vi "TicTacToe.vi"() -> ()   [LabVIEW 2018]
panel:
  out "Human Win":dbl
  in  "Show XO plate":bool
  out "Computer Win":dbl
  out "Tie":bool
  out "No one Won":bool
  out "Game Over":bool
  out "Computer Won":bool
  out "Human Won":bool
  out "Turn":string
  out "XO array":string[][](array[string])
  in  "START GAME":bool
  in  "Boolean 9":bool
  in  "Boolean 8":bool
  in  "Boolean 7":bool
  in  "Boolean 6":bool
  in  "Boolean 5":bool
  in  "Boolean 4":bool
  in  "Boolean 3":bool
  in  "Boolean 2":bool
  in  "Boolean":bool
  in  "STOP GAME":bool
  in  "Turn":bool
  # "XO GAME"
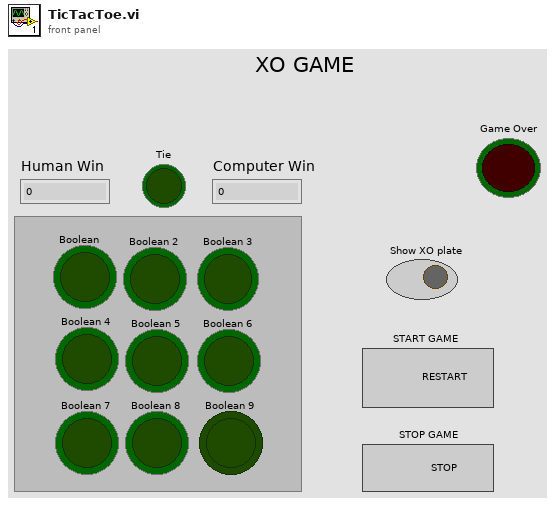
[diagram p1: front panel]
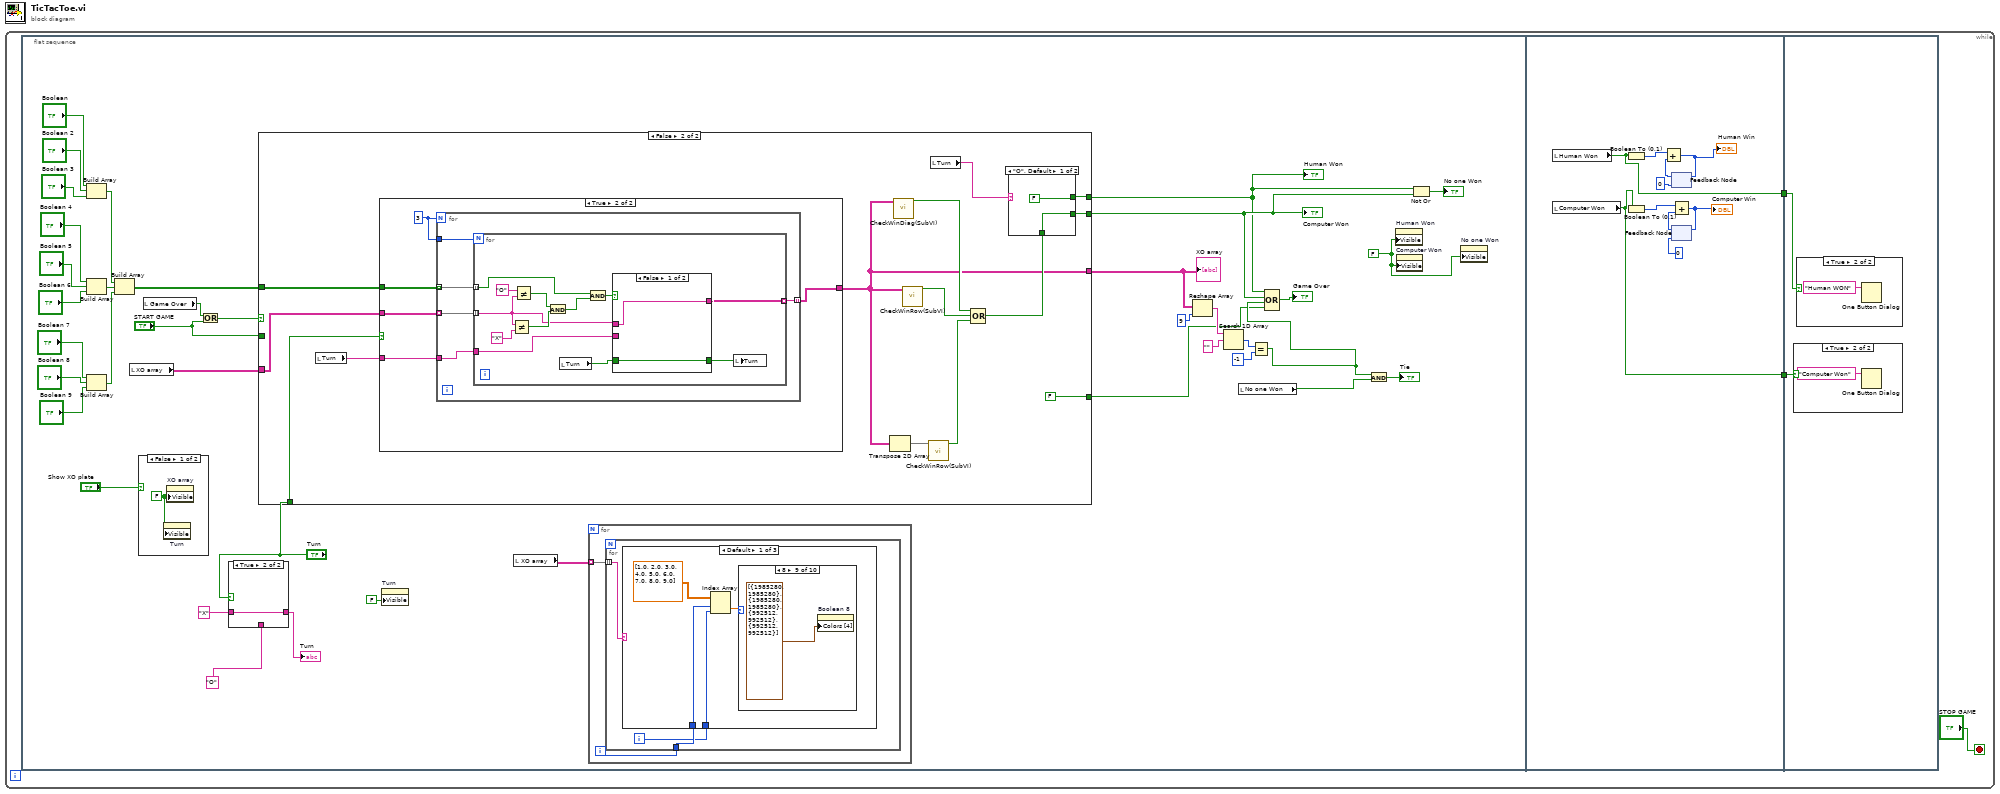
[diagram p0: block diagram]
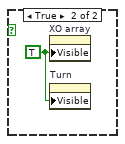
[diagram p2: hidden frame]
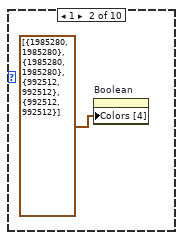
[diagram p4: hidden frame]
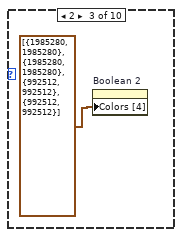
[diagram p5: hidden frame]
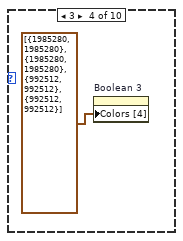
[diagram p6: hidden frame]
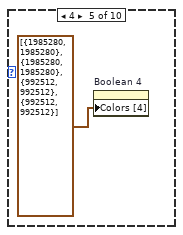
[diagram p7: hidden frame]
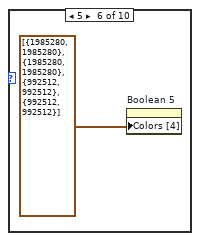
[diagram p8: hidden frame]
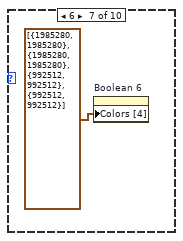
[diagram p9: hidden frame]
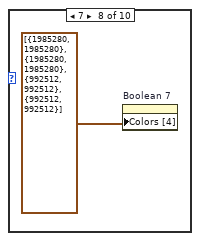
[diagram p10: hidden frame]
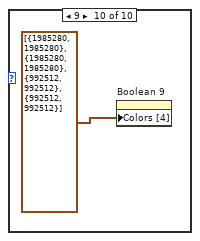
[diagram p11: hidden frame]
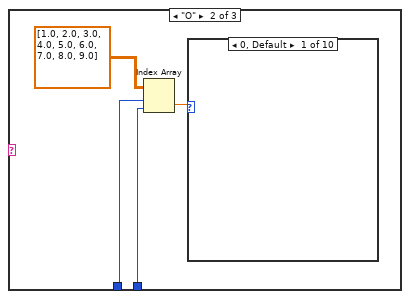
[diagram p12: hidden frame]
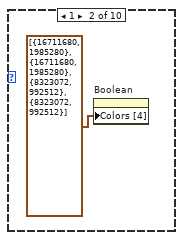
[diagram p13: hidden frame]
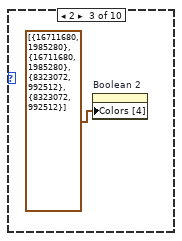
[diagram p14: hidden frame]
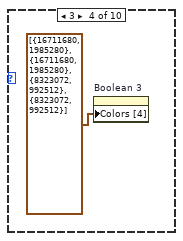
[diagram p15: hidden frame]
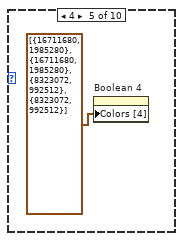
[diagram p16: hidden frame]
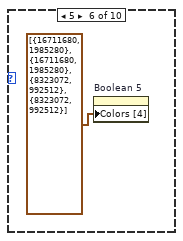
[diagram p17: hidden frame]
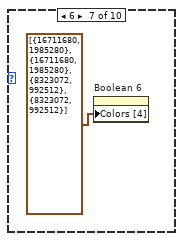
[diagram p18: hidden frame]
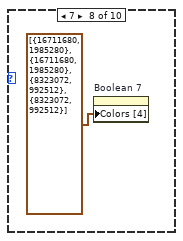
[diagram p19: hidden frame]
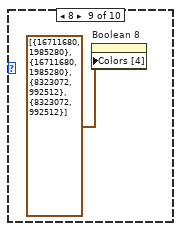
[diagram p20: hidden frame]
diagram:
  n1 = while {
    stop <- "STOP GAME" stop-if-true
    n2 = flat-sequence {
      tunnel: [w156] -> w2
      tunnel: [w155] -> w1
      tunnel: w2 -> [w166]
      tunnel: w1 -> [w165]
      frame #0 {
        w5 = FALSE ("Visible")
        n3 = Build Array("Boolean", "Boolean 2", "Boolean 3") -> (w40:bool[])
        n4 = Build Array("Boolean 4", "Boolean 5", "Boolean 6") -> (w41:bool[])
        n5 = Build Array("Boolean 7", "Boolean 8", "Boolean 9") -> (w42:bool[])
        n6 = Build Array(w40, w41, w42) -> (w32:bool[][])
        n7 = local read "XO array"() -> (w31:string[][])
        n8 = case shown="False" "Show XO plate" {
          frame False {
            w43 = FALSE ("Visible")
            n9 = property on="Turn" class="Str"("Visible"=w43) -> ()  [unwired: 2 in, 2 out]
            n10 = property on="XO array" class="Arr (strict)"("Visible"=w43) -> ()  [unwired: 2 in, 2 out]
          }
          frame True {
            w44 = TRUE ("Visible")
            n11 = property on="XO array" class="Arr (strict)"("Visible"=w44) -> ()  [unwired: 2 in, 2 out]
            n12 = property on="Turn" class="Str"("Visible"=w44) -> ()  [unwired: 2 in, 2 out]
          }
        }
        n13 = local read "Game Over"() -> (w24:bool)
        n14 = Or(x=w24, y="START GAME") -> (x .or. y?=w23:bool)
        n15 = case shown="True" "Turn" {
          tunnel: "X" -> [_ w90]
          tunnel: [w89 w90] -> w29
          tunnel: "O" ("x") -> [w89 _]
          frame False {
          }
          frame True {
          }
        }
        "Turn" <- w29
        n16 = case shown="False" w23 {
          tunnel: w32 -> [_ w119]
          tunnel: w31 -> [w95 w118]
          tunnel: "Turn" -> [_ w116]
          tunnel: "START GAME" -> [w96 _]
          tunnel: [w94 w109] -> w7
          tunnel: [w93 w108] -> w6
          tunnel: [w92 w107] -> w11
          tunnel: [w91 FALSE] -> w4
          frame True {
            n17 = case shown="True" w96 {
              tunnel: [w99 w104] -> w92
              tunnel: [w98 w103] -> w93
              tunnel: [w98 w103] -> w94
              tunnel: w95 -> [w99 _]
              tunnel: [TRUE FALSE] -> w91
              frame False {
                w98 = FALSE
              }
              frame True {
                w101 = FALSE
                w103 = FALSE
                w102 = 3
                n18 = local write "Boolean"(w101) -> ()
                n19 = local write "Boolean 2"(w101) -> ()
                n20 = local write "Boolean 3"(w101) -> ()
                n21 = local write "Boolean 6"(w101) -> ()
                n22 = local write "Boolean 5"(w101) -> ()
                n23 = local write "Boolean 7"(w101) -> ()
                n24 = local write "Boolean 8"(w101) -> ()
                n25 = local write "Boolean 9"(w101) -> ()
                n26 = local write "Boolean 4"(w101) -> ()
                n27 = Initialize Array("", w102, w102) -> (w104:string[][])
              }
            }
          }
          frame False {
            n28 = local read "Turn"() -> (w117:string)
            n29 = case shown="True" w116 {
              tunnel: w119 -> [_ w132]
              tunnel: w118 -> [w126 w130]
              tunnel: [w127 w129] -> w107
              tunnel: w117 -> [_ w128]
              frame False {
                n30 = local read "Turn"() -> (w125:bool)
                n31 = call "AI algorithm(SubVI).vi"("Turn"=w125, "XO array"=w126) -> ("Turn 2"=w124:bool, "XO array 2"=w127:string[][])
                n32 = local write "Turn"(w124) -> ()
              }
              frame True {
                w131 = 3
                n33 = for {
                  N: w131 -> [_]
                  tunnel: w131 -> [w137]
                  tunnel: w132 -> [w136] mode=indexing
                  tunnel: w130 -> [w135] mode=indexing
                  tunnel: [w134] -> w129 mode=indexing
                  tunnel: w128 -> [w133]
                  n34 = for {
                    N: w137 -> [_]
                    tunnel: w136 -> [w145] mode=indexing
                    tunnel: w135 -> [w142] mode=indexing
                    tunnel: w133 -> [w140]
                    tunnel: [w141] -> w134 mode=indexing
                    n35 = Not Equal?(x=w142, y="X") -> (x != y?=w146:bool)
                    n36 = Not Equal?(x="O", y=w142) -> (x != y?=w147:bool)
                    n37 = And(x=w147, y=w146) -> (x .and. y?=w144:bool)
                    n38 = local read "Turn"() -> (w138:bool)
                    n39 = And(x=w145, y=w144) -> (x .and. y?=w143:bool)
                    n40 = case shown="False" w143 {
                      tunnel: w142 -> [w151 _]
                      tunnel: [w151 w152] -> w141
                      tunnel: w140 -> [_ w152]
                      tunnel: [w150 w153] -> w139
                      tunnel: w138 -> [w150 w154]
                      frame False {
                      }
                      frame True {
                        n41 = Not(x=w154) -> (.not. x?=w153:bool)
                      }
                    }
                    n42 = local write "Turn"(w139) -> ()
                  }
                }
              }
            }
            n43 = Transpose 2D Array(2D array=w107) -> (transposed array=w115:string[][])
            n44 = call "CheckWinDiag(SubVI).vi"("Array"=w107) -> ("x .or. y?"=w114:bool)  [unwired: 10 in]
            n45 = call "CheckWinRow(SubVI).vi"("Array"=w107) -> ("x .or. y? 2"=w113:bool)  [unwired: 10 in]
            n46 = call "CheckWinRow(SubVI).vi"("Array"=w115) -> ("x .or. y? 2"=w112:bool)  [unwired: 10 in]
            n47 = local read "Turn"() -> (w110:string)
            n48 = Compound Arithmetic op=OR(w114, w113, w112) -> (w111:bool)
            n49 = case shown="\"O\", Default" w110 {
              tunnel: w111 -> [w121 w122]
              tunnel: [w121 FALSE] -> w109
              tunnel: [FALSE w122] -> w108
              frame "O", Default {
              }
              frame "X" {
              }
            }
          }
        }
        "Human Won" <- w6
        "Computer Won" <- w7
        "XO array" <- w11
        n50 = property on="Turn" class="Bool (strict)"("Visible"=FALSE) -> ()  [unwired: 2 in, 2 out]
        n51 = local read "XO array"() -> (w10:string[][])
        n52 = for {
          tunnel: w10 -> [w45] mode=indexing
          i -> [w46]
          n53 = for {
            tunnel: w46 -> [w49]
            tunnel: w45 -> [w47] mode=indexing
            i -> [w48]
            n54 = case shown="Default" w47 {
              tunnel: w49 -> [w53 w64 w77]
              tunnel: w48 -> [w52 w63 w78]
              frame Default {
                n55 = Index Array(array=dbl[][] [[1.0, 2.0, 3.0], [4.0, 5.0, 6.0], [7.0, 8.0, 9.0]] ("Array"), index (row)=w53, index (col)=w52) -> (element=w50:dbl)
                n56 = case shown="8" w50 {
                  frame 0, Default {
                  }
                  frame 1 {
                    n57 = property on="Boolean" class="Bool (strict)"("Colors [4]"=cluster{u32, u32}[] [{1985280, 1985280}, {1985280, 1985280}, {992512, 992512}, {992512, 992512}]) -> ()  [unwired: 2 in, 2 out]
                  }
                  frame 2 {
                    n58 = property on="Boolean 2" class="Bool (strict)"("Colors [4]"=cluster{u32, u32}[] [{1985280, 1985280}, {1985280, 1985280}, {992512, 992512}, {992512, 992512}]) -> ()  [unwired: 2 in, 2 out]
                  }
                  frame 3 {
                    n59 = property on="Boolean 3" class="Bool (strict)"("Colors [4]"=cluster{u32, u32}[] [{1985280, 1985280}, {1985280, 1985280}, {992512, 992512}, {992512, 992512}]) -> ()  [unwired: 2 in, 2 out]
                  }
                  frame 4 {
                    n60 = property on="Boolean 4" class="Bool (strict)"("Colors [4]"=cluster{u32, u32}[] [{1985280, 1985280}, {1985280, 1985280}, {992512, 992512}, {992512, 992512}]) -> ()  [unwired: 2 in, 2 out]
                  }
                  frame 5 {
                    n61 = property on="Boolean 5" class="Bool (strict)"("Colors [4]"=cluster{u32, u32}[] [{1985280, 1985280}, {1985280, 1985280}, {992512, 992512}, {992512, 992512}]) -> ()  [unwired: 2 in, 2 out]
                  }
                  frame 6 {
                    n62 = property on="Boolean 6" class="Bool (strict)"("Colors [4]"=cluster{u32, u32}[] [{1985280, 1985280}, {1985280, 1985280}, {992512, 992512}, {992512, 992512}]) -> ()  [unwired: 2 in, 2 out]
                  }
                  frame 7 {
                    n63 = property on="Boolean 7" class="Bool (strict)"("Colors [4]"=cluster{u32, u32}[] [{1985280, 1985280}, {1985280, 1985280}, {992512, 992512}, {992512, 992512}]) -> ()  [unwired: 2 in, 2 out]
                  }
                  frame 8 {
                    n64 = property on="Boolean 8" class="Bool (strict)"("Colors [4]"=cluster{u32, u32}[] [{1985280, 1985280}, {1985280, 1985280}, {992512, 992512}, {992512, 992512}]) -> ()  [unwired: 2 in, 2 out]
                  }
                  frame 9 {
                    n65 = property on="Boolean 9" class="Bool (strict)"("Colors [4]"=cluster{u32, u32}[] [{1985280, 1985280}, {1985280, 1985280}, {992512, 992512}, {992512, 992512}]) -> ()  [unwired: 2 in, 2 out]
                  }
                }
              }
              frame "O" {
                n66 = Index Array(array=dbl[][] [[1.0, 2.0, 3.0], [4.0, 5.0, 6.0], [7.0, 8.0, 9.0]] ("Array"), index (row)=w64, index (col)=w63) -> (element=w65:dbl)
                n67 = case shown="0, Default" w65 {
                  frame 0, Default {
                  }
                  frame 1 {
                    n68 = property on="Boolean" class="Bool (strict)"("Colors [4]"=cluster{u32, u32}[] [{16711680, 1985280}, {16711680, 1985280}, {8323072, 992512}, {8323072, 992512}]) -> ()  [unwired: 2 in, 2 out]
                  }
                  frame 2 {
                    n69 = property on="Boolean 2" class="Bool (strict)"("Colors [4]"=cluster{u32, u32}[] [{16711680, 1985280}, {16711680, 1985280}, {8323072, 992512}, {8323072, 992512}]) -> ()  [unwired: 2 in, 2 out]
                  }
                  frame 3 {
                    n70 = property on="Boolean 3" class="Bool (strict)"("Colors [4]"=cluster{u32, u32}[] [{16711680, 1985280}, {16711680, 1985280}, {8323072, 992512}, {8323072, 992512}]) -> ()  [unwired: 2 in, 2 out]
                  }
                  frame 4 {
                    n71 = property on="Boolean 4" class="Bool (strict)"("Colors [4]"=cluster{u32, u32}[] [{16711680, 1985280}, {16711680, 1985280}, {8323072, 992512}, {8323072, 992512}]) -> ()  [unwired: 2 in, 2 out]
                  }
                  frame 5 {
                    n72 = property on="Boolean 5" class="Bool (strict)"("Colors [4]"=cluster{u32, u32}[] [{16711680, 1985280}, {16711680, 1985280}, {8323072, 992512}, {8323072, 992512}]) -> ()  [unwired: 2 in, 2 out]
                  }
                  frame 6 {
                    n73 = property on="Boolean 6" class="Bool (strict)"("Colors [4]"=cluster{u32, u32}[] [{16711680, 1985280}, {16711680, 1985280}, {8323072, 992512}, {8323072, 992512}]) -> ()  [unwired: 2 in, 2 out]
                  }
                  frame 7 {
                    n74 = property on="Boolean 7" class="Bool (strict)"("Colors [4]"=cluster{u32, u32}[] [{16711680, 1985280}, {16711680, 1985280}, {8323072, 992512}, {8323072, 992512}]) -> ()  [unwired: 2 in, 2 out]
                  }
                  frame 8 {
                    n75 = property on="Boolean 8" class="Bool (strict)"("Colors [4]"=cluster{u32, u32}[] [{16711680, 1985280}, {16711680, 1985280}, {8323072, 992512}, {8323072, 992512}]) -> ()  [unwired: 2 in, 2 out]
                  }
                  frame 9 {
                    n76 = property on="Boolean 9" class="Bool (strict)"("Colors [4]"=cluster{u32, u32}[] [{16711680, 1985280}, {16711680, 1985280}, {8323072, 992512}, {8323072, 992512}]) -> ()  [unwired: 2 in, 2 out]
                  }
                }
              }
              frame "X" {
                n77 = Index Array(array=dbl[][] [[1.0, 2.0, 3.0], [4.0, 5.0, 6.0], [7.0, 8.0, 9.0]] ("Array"), index (row)=w77, index (col)=w78) -> (element=w79:dbl)
                n78 = case shown="1" w79 {
                  frame 0, Default {
                  }
                  frame 1 {
                    n79 = property on="Boolean" class="Bool (strict)"("Colors [4]"=cluster{u32, u32}[] [{6618880, 6618880}, {6618880, 6618880}, {3309312, 3309312}, {3309312, 3309312}]) -> ()  [unwired: 2 in, 2 out]
                  }
                  frame 2 {
                    n80 = property on="Boolean 2" class="Bool (strict)"("Colors [4]"=cluster{u32, u32}[] [{6618880, 6618880}, {6618880, 6618880}, {3309312, 3309312}, {3309312, 3309312}]) -> ()  [unwired: 2 in, 2 out]
                  }
                  frame 3 {
                    n81 = property on="Boolean 3" class="Bool (strict)"("Colors [4]"=cluster{u32, u32}[] [{6618880, 6618880}, {6618880, 6618880}, {3309312, 3309312}, {3309312, 3309312}]) -> ()  [unwired: 2 in, 2 out]
                  }
                  frame 4 {
                    n82 = property on="Boolean 4" class="Bool (strict)"("Colors [4]"=cluster{u32, u32}[] [{6618880, 6618880}, {6618880, 6618880}, {3309312, 3309312}, {3309312, 3309312}]) -> ()  [unwired: 2 in, 2 out]
                  }
                  frame 5 {
                    n83 = property on="Boolean 5" class="Bool (strict)"("Colors [4]"=cluster{u32, u32}[] [{6618880, 6618880}, {6618880, 6618880}, {3309312, 3309312}, {3309312, 3309312}]) -> ()  [unwired: 2 in, 2 out]
                  }
                  frame 6 {
                    n84 = property on="Boolean 6" class="Bool (strict)"("Colors [4]"=cluster{u32, u32}[] [{6618880, 6618880}, {6618880, 6618880}, {3309312, 3309312}, {3309312, 3309312}]) -> ()  [unwired: 2 in, 2 out]
                  }
                  frame 7 {
                    n85 = property on="Boolean 7" class="Bool (strict)"("Colors [4]"=cluster{u32, u32}[] [{6618880, 6618880}, {6618880, 6618880}, {3309312, 3309312}, {3309312, 3309312}]) -> ()  [unwired: 2 in, 2 out]
                  }
                  frame 8 {
                    n86 = property on="Boolean 8" class="Bool (strict)"("Colors [4]"=cluster{u32, u32}[] [{6618880, 6618880}, {6618880, 6618880}, {3309312, 3309312}, {3309312, 3309312}]) -> ()  [unwired: 2 in, 2 out]
                  }
                  frame 9 {
                    n87 = property on="Boolean 9" class="Bool (strict)"("Colors [4]"=cluster{u32, u32}[] [{6618880, 6618880}, {6618880, 6618880}, {3309312, 3309312}, {3309312, 3309312}]) -> ()  [unwired: 2 in, 2 out]
                  }
                }
              }
            }
          }
        }
        n88 = Reshape Array(w11, 9 ("dimension size")) -> (w17:string[])
        n89 = Search 1D Array(1D array=w17, element="") -> (index of element=w15:i32)  [unwired: 1 in]
        n90 = local read "No one Won"() -> (w19:bool)
        n91 = Equal?(x=w15, y=-1) -> (x = y?=w12:bool)
        n92 = Compound Arithmetic op=OR(w6, w7, w12, w4) -> (→"Game Over":bool)
        n93 = And(x=w12, y=w19) -> (x .and. y?=→"Tie":bool)
        n94 = property on="Human Won" class="Bool (strict)"("Visible"=w5) -> ()  [unwired: 2 in, 2 out]
        n95 = property on="Computer Won" class="Bool (strict)"("Visible"=w5) -> ()  [unwired: 2 in, 2 out]
        n96 = Not Or(1:w7, 2:w6) -> (0:→"No one Won":bool)
        n97 = property on="No one Won" class="Bool (strict)"("Visible"=w5) -> ()  [unwired: 2 in, 2 out]
      }
      frame #1 {
        n98 = local read "Human Won"() -> (w155:bool)
        n99 = local read "Computer Won"() -> (w156:bool)
        n100 = Boolean To (0,1)(Boolean=w155) -> (0, 1=w159:i16)
        n101 = Boolean To (0,1)(Boolean=w156) -> (0, 1=w157:i16)
        n102 = feedback #1(i16 0) -> (w160:i16)
        n103 = Add(x=w159, y=w160) -> (x+y=w162:i16)
        "Human Win" <- w162
        n104 = feedback-in #1(w162) -> ()
        n105 = feedback #2(i16 0) -> (w158:i16)
        n106 = Add(x=w157, y=w158) -> (x+y=w161:i16)
        "Computer Win" <- w161
        n107 = feedback-in #2(w161) -> ()
      }
      frame #2 {
        n108 = case shown="True" w166 {
          frame False {
          }
          frame True {
            n109 = One Button Dialog(message="Computer Won") -> ()  [unwired: 1 in, 1 out]
          }
        }
        n110 = case shown="True" w165 {
          frame False {
          }
          frame True {
            n111 = One Button Dialog(message="Human WON") -> ()  [unwired: 1 in, 1 out]
          }
        }
      }
    }
  }
